vi "ICM Close.vi"(0 "ICM Ref":refnum<class "Modbus Master.lvclass">, 11 "error in (no error)":errorcluster) -> (15 "error out":errorcluster)   [LabVIEW 2024]
doc: "Close the serial modbus connection to the ICM 4.0 module."
uses:
  <vilib>/NI/Modbus Library/API/Master/Modbus Master.lvclass
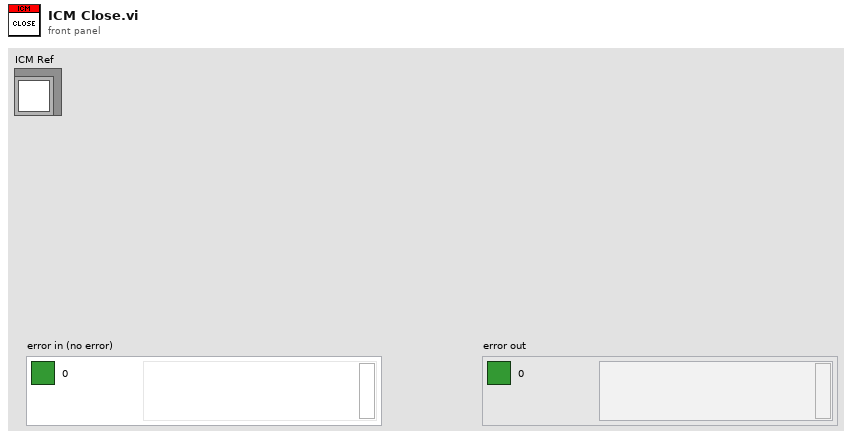
[diagram p1: front panel]
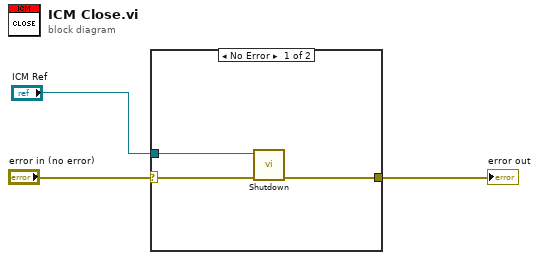
[diagram p0: block diagram]
diagram:
  n1 = case shown="No Error" "error in (no error)" {
    selector: "error in (no error)" -> [w6 w7]
    tunnel: [w5 w7] -> w2
    tunnel: "ICM Ref" -> [w4 _]
    frame No Error {
      n2 = call-dynamic "Shutdown.vi"("error in"=w6, "Modbus master in"=w4) -> ("error out"=w5:errorcluster)  [unwired: 9 in]
    }
    frame Error {
    }
  }
  "error out" <- w2
